vi "NiXnet ConvertByteArrayToFramesSinglePoint.vi"(6 "contextId":T1, 8 "error in":errorcluster, 9 "timeout (ms)":i32=-1, 10 "Request Data":T4, 11 "gRPC ID":T1) -> (0 "error out":errorcluster, 2 "Response Data":T2, 3 "gRPC ID out":T1)   [LabVIEW 2025, in "xnet-grpc_client.lvlib"]
uses:
  xnet-grpc_client.lvlib
  <vilib>/gRPC/LabVIEW gRPC Library/Shared/grpcId.ctl
  RPC Messages/nixnet_grpc_ConvertByteArrayToFramesSinglePointRequest.ctl
  RPC Messages/nixnet_grpc_ConvertByteArrayToFramesSinglePointRequest_protocol_enum/nixnet_grpc_ConvertByteArrayToFramesSinglePointRequest_protocol_enum.lvclass
  RPC Messages/nidevice_grpc_Session.ctl
  RPC Messages/nixnet_grpc_ConvertByteArrayToFramesSinglePointResponse.ctl
  RPC Messages/nixnet_grpc_FrameBufferResponse.ctl
  RPC Messages/nixnet_grpc_FrameBufferResponse_frame/nixnet_grpc_FrameBufferResponse_frame.lvclass
  RPC Messages/nixnet_grpc_ConvertByteArrayToFramesSinglePointResponse_Flat.ctl
  RPC Messages/nixnet_grpc_FrameBufferResponse_Flat.ctl
  RPC Messages/nixnet_grpc_FrameResponse_Flat.ctl
  RPC Messages/nixnet_grpc_FrameType.ctl
  RPC Messages/nixnet_grpc_FrameFlags.ctl
  RPC Messages/nixnet_grpc_EnetFrameResponse_Flat.ctl
  RPC Messages/nixnet_grpc_EnetFrameType.ctl
  RPC Messages/nixnet_grpc_EnetFlags.ctl
  RPC Messages/nixnet_grpc_ConvertByteArrayToFramesSinglePointRequest_protocol_enum/nixnet_grpc_ConvertByteArrayToFramesSinglePointRequest_protocol_enum.lvclass/nixnet_grpc_ConvertByteArrayToFramesSinglePointRequest_protocol_enum.ctl
  RPC Messages/nixnet_grpc_FrameBufferResponse_frame/nixnet_grpc_FrameBufferResponse_frame.lvclass/nixnet_grpc_FrameBufferResponse_frame.ctl
  14035477-4c25-4107-8ed5-d0c4ef420ce5.vi
  RPC Messages/RichToFlatnidevice_grpc_Session.vi
  RPC Messages/nixnet_grpc_ConvertByteArrayToFramesSinglePointRequest_protocol_enum/GetActiveFieldIndex.vi
  RPC Messages/nixnet_grpc_ConvertByteArrayToFramesSinglePointRequest_protocol_enum/Getprotocol.vi
  RPC Messages/nixnet_grpc_ConvertByteArrayToFramesSinglePointRequest_protocol_enum/Getprotocol_raw.vi
  <vilib>/gRPC/LabVIEW gRPC Library/Shared/TranslateGrpcError.vi
  <vilib>/gRPC/LabVIEW gRPC Library/Shared/Wait On Occurrence Wrapper.vi
  RPC Messages/FlatToRichnixnet_grpc_FrameBufferResponse.vi
  <vilib>/gRPC/LabVIEW gRPC Library/Shared/Wait On Occurence.vi
  RPC Messages/nixnet_grpc_FrameBufferResponse_frame/Setcan.vi
  RPC Messages/FlatToRichnixnet_grpc_FrameResponse.vi
  RPC Messages/nixnet_grpc_FrameBufferResponse_frame/Setlin.vi
  RPC Messages/nixnet_grpc_FrameBufferResponse_frame/Setflex_ray.vi
  RPC Messages/nixnet_grpc_FrameBufferResponse_frame/Setj1939.vi
  RPC Messages/nixnet_grpc_FrameBufferResponse_frame/Setenet.vi
  RPC Messages/FlatToRichnixnet_grpc_EnetFrameResponse.vi
  <vilib>/gRPC/LabVIEW gRPC Library/Server API/Server/Get Server DLL Path.vi
  <vilib>/Utility/error.llb/Error Cluster From Error Code.vi
  <vilib>/Utility/config.llb/Open Config Data.vi
  <vilib>/Utility/config.llb/Write Key.vi
  <vilib>/Utility/config.llb/Write Key (Boolean).vi
  <vilib>/Utility/config.llb/Not A Config Data Refnum.vi
  <vilib>/Utility/config.llb/Read Key.vi
  <vilib>/Utility/config.llb/Read Key (Boolean).vi
  <vilib>/Utility/config.llb/Close Config Data.vi
  RPC Messages/nixnet_grpc_FrameBufferResponse_frame/GetActiveFieldName.vi
  <vilib>/gRPC/LabVIEW gRPC Library/grpc-lvsupport-release.lvlib
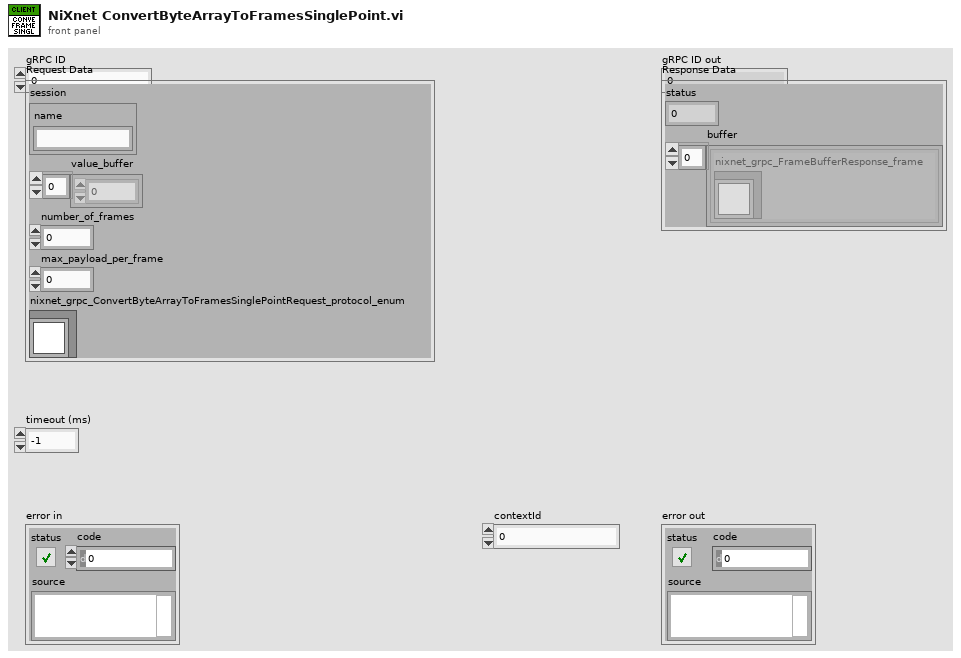
[diagram p1: front panel]
types:
  T1 = typedef "grpc-lvsupport-release.lvlib/grpcId.ctl" = u64
  T2 = typedef "xnet-grpc_client.lvlib/nixnet_grpc_ConvertByteArrayToFramesSinglePointResponse.ctl" = cluster{"status":i32, "buffer":T3[]}
  T3 = typedef "xnet-grpc_client.lvlib/nixnet_grpc_FrameBufferResponse.ctl" = cluster{"nixnet_grpc_FrameBufferResponse_frame":refnum<class "nixnet_grpc_FrameBufferResponse_frame.lvclass">}
  T4 = typedef "xnet-grpc_client.lvlib/nixnet_grpc_ConvertByteArrayToFramesSinglePointRequest.ctl" = cluster{"session":T5, "value_buffer":u8[], "number_of_frames":u32, "max_payload_per_frame":u32, "nixnet_grpc_ConvertByteArrayToFramesSinglePointRequest_protocol_enum":refnum<class "nixnet_grpc_ConvertByteArrayToFramesSinglePointRequest_protocol_enum.lvclass">}
  T5 = typedef "xnet-grpc_client.lvlib/nidevice_grpc_Session.ctl" = cluster{"name":string}
  T6 = typedef "xnet-grpc_client.lvlib/nixnet_grpc_ConvertByteArrayToFramesSinglePointResponse_Flat.ctl" = cluster{"status":i32, "buffer":T7[]}
  T7 = typedef "xnet-grpc_client.lvlib/nixnet_grpc_FrameBufferResponse_Flat.ctl" = cluster{"nixnet_grpc_FrameBufferResponse_frame_selected_index":i32, "can":T8, "lin":T8, "flex_ray":T8, "j1939":T8, "enet":T11}
  T8 = typedef "xnet-grpc_client.lvlib/nixnet_grpc_FrameResponse_Flat.ctl" = cluster{"timestamp":u64, "identifier":u32, "type":T9, "type_raw":u32, "flags":T10[], "flags_raw":u32, "info":u32, "payload":u8[]}
  T9 = typedef "xnet-grpc_client.lvlib/nixnet_grpc_FrameType.ctl" = enum32{"FRAME_TYPE_CAN_DATA", "FRAME_TYPE_CAN_REMOTE", "FRAME_TYPE_CAN_BUS_ERROR", "FRAME_TYPE_CAN20_DATA", "FRAME_TYPE_CANFD_DATA", "FRAME_TYPE_CANFDBRS_DATA", "FRAME_TYPE_FLEX_RAY_DATA", "FRAME_TYPE_FLEX_RAY_NULL", "FRAME_TYPE_FLEX_RAY_SYMBOL", "FRAME_TYPE_LIN_DATA", "FRAME_TYPE_LIN_BUS_ERROR", "FRAME_TYPE_LIN_NO_RESPONSE", "FRAME_TYPE_J1939_DATA", "FRAME_TYPE_SPECIAL_DELAY", "FRAME_TYPE_SPECIAL_LOG_TRIGGER", "FRAME_TYPE_SPECIAL_START_TRIGGER"}
  T10 = typedef "xnet-grpc_client.lvlib/nixnet_grpc_FrameFlags.ctl" = enum32{"FRAME_FLAGS_UNSPECIFIED", "FRAME_FLAGS_FLEX_RAY_STARTUP", "FRAME_FLAGS_FLEX_RAY_SYNC", "FRAME_FLAGS_FLEX_RAY_PREAMBLE", "FRAME_FLAGS_FLEX_RAY_CH_A", "FRAME_FLAGS_FLEX_RAY_CH_B", "FRAME_FLAGS_LIN_EVENT_SLOT", "FRAME_FLAGS_TRANSMIT_ECHO"}
  T11 = typedef "xnet-grpc_client.lvlib/nixnet_grpc_EnetFrameResponse_Flat.ctl" = cluster{"type":T12, "type_raw":u32, "device_timestamp":u64, "network_timestamp":u64, "flags_mapped":T13[], "flags_raw":u32, "frame_data":u8[]}
  T12 = typedef "xnet-grpc_client.lvlib/nixnet_grpc_EnetFrameType.ctl" = enum32{"ENET_FRAME_TYPE_DATA", "ENET_FRAME_TYPE_DELAY", "ENET_FRAME_TYPE_FUTURE_TIME_WAIT"}
  T13 = typedef "xnet-grpc_client.lvlib/nixnet_grpc_EnetFlags.ctl" = enum32{"ENET_FLAGS_UNSPECIFIED", "ENET_FLAGS_TRANSMIT", "ENET_FLAGS_RECEIVE", "ENET_FLAGS_NETWORK_SYNCED", "ENET_FLAGS_ERROR"}
  T14 = typedef "xnet-grpc_client.lvlib/nixnet_grpc_ConvertByteArrayToFramesSinglePointRequest_Flat.ctl" = cluster{"session":T15, "value_buffer":u8[], "number_of_frames":u32, "max_payload_per_frame":u32, "nixnet_grpc_ConvertByteArrayToFramesSinglePointRequest_protocol_enum_selected_index":i32, "protocol":T16, "protocol_raw":u32}
  T15 = typedef "xnet-grpc_client.lvlib/nidevice_grpc_Session_Flat.ctl" = cluster{"name":string}
  T16 = typedef "xnet-grpc_client.lvlib/nixnet_grpc_Protocol.ctl" = enum32{"PROTOCOL_UNSPECIFIED", "PROTOCOL_CAN", "PROTOCOL_LIN", "PROTOCOL_FLEX_RAY", "PROTOCOL_J1939", "PROTOCOL_ENET"}
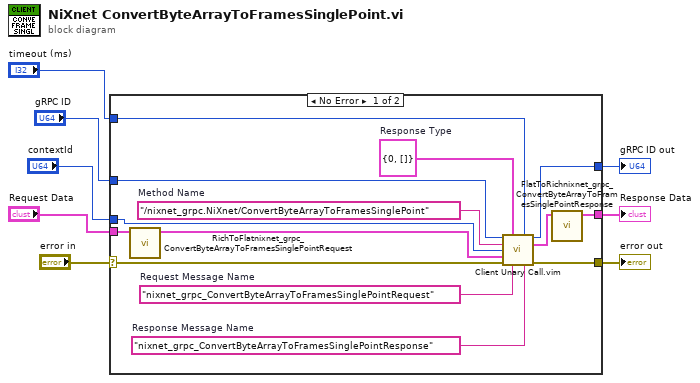
[diagram p0: block diagram]
diagram:
  n1 = case shown="No Error" "error in" {
    selector: "error in" -> [w18 w23]
    tunnel: [w17 w23] -> w7
    tunnel: "gRPC ID" -> [w16 w24]
    tunnel: [w15 w24] -> w5
    tunnel: "Request Data" -> [w12 _]
    tunnel: [w9 _] -> w3
    tunnel: "timeout (ms)" -> [w14 _]
    tunnel: "contextId" -> [w13 _]
    frame No Error {
      w19 = "nixnet_grpc_ConvertByteArrayToFramesSinglePointResponse"  # Response Message Name
      w20 = "nixnet_grpc_ConvertByteArrayToFramesSinglePointRequest"  # Request Message Name
      w21 = T6 {"status"=0, "buffer"=[]}  # Response Type
      w22 = "/nixnet_grpc.NiXnet/ConvertByteArrayToFramesSinglePoint"  # Method Name
      n2 = call "RichToFlatnixnet_grpc_ConvertByteArrayToFramesSinglePointRequest.vi"("InputCluster"=w12) -> ("OutputCluster"=w11:T14)  [unwired: 10 in]
      n3 = call "Client Unary Call.vim"("ClientID in"=w16, "Response Type"=w21, "timeout (ms)"=w14, "Method Name"=w22, "contextId"=w13, "Request Data"=w11, "error in"=w18, "Request Message Name"=w20, "Response Message Name"=w19) -> ("ClientID out"=w15:u64, "Response Data"=w10:T6, "error out"=w17:errorcluster)  [unwired: 4 in]
      n4 = call "FlatToRichnixnet_grpc_ConvertByteArrayToFramesSinglePointResponse.vi"("InputCluster"=w10) -> ("OutputCluster"=w9:T2)  [unwired: 10 in]
    }
    frame Error {
    }
  }
  "error out" <- w7
  "gRPC ID out" <- w5
  "Response Data" <- w3
